vi "Write Height.vi"(8 "error in (no error)":errorcluster, 10 "Height":u32=250, 11 "2D Plot.lvclass in":refnum<class "2D Plot.lvclass">) -> (0 "error out":errorcluster, 3 "2D Plot.lvclass out":refnum<class "2D Plot.lvclass">)   [LabVIEW 2020, in "2D Plot.lvclass"]
uses:
  <vilib>/Math Plots/2D Math Plots/2D Plot/2D Plot/2D Plot.lvclass
  <vilib>/Math Plots/2D Math Plots/2D Plot/2D Plot/2D Plot.lvclass/2D Plot.ctl
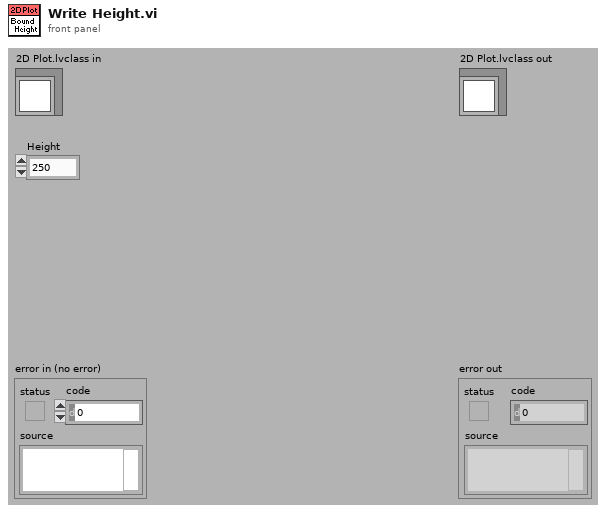
[diagram p1: front panel]
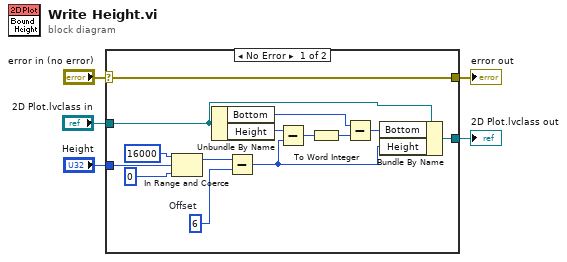
[diagram p0: block diagram]
diagram:
  n1 = case shown="No Error" "error in (no error)" {
    selector: "error in (no error)" -> [w19 w20]
    tunnel: [w19 w20] -> w4
    tunnel: [w18 w21] -> w2
    tunnel: "2D Plot.lvclass in" -> [w13 w21]
    tunnel: "Height" -> [w7 _]
    frame No Error {
      w11 = u32 6  # Offset
      n2 = In Range and Coerce(upper limit=u32 16000, x=w7, lower limit=u32 0) -> (coerced(x)=w6:u32)  [unwired: 1 out]
      n3 = Unbundle By Name(w13) -> ("Bottom"=w17:i16, "Height"=w14:u32)
      n4 = Subtract(x=w6, y=w11) -> (x-y=w10:u32)
      n5 = Subtract(x=w14, y=w10) -> (x-y=w15:u32)
      n6 = To Word Integer(number=w15) -> (16bit integer=w16:i16)
      n7 = Subtract(x=w17, y=w16) -> (x-y=w12:i16)
      n8 = Bundle By Name(cluster=w13, "Bottom"=w12, "Height"=w10) -> (w18:refnum<class "2D Plot.lvclass">)
    }
    frame Error {
    }
  }
  "error out" <- w4
  "2D Plot.lvclass out" <- w2
